vi "GeoCal_RangeWalk_process.vi"(0 "Position":string) -> (7 "Boolean":bool=TRUE)   [LabVIEW 2018]
panel:
  in  "Acquire":bool
  # "Geo Cal & Range Walk Test"
  # "please make sure the robot is in position\n                 then press the Acquire button"
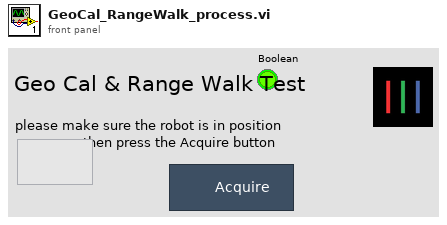
[diagram p1: front panel]
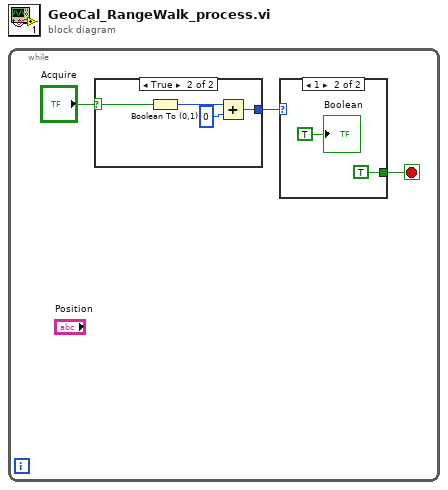
[diagram p0: block diagram]
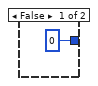
[diagram p2: hidden frame]
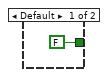
[diagram p3: hidden frame]
diagram:
  n1 = while {
    stop <- w3 stop-if-true
    n2 = case shown="True" "Acquire" {
      selector: "Acquire" -> [_ w5]
      tunnel: [i16 0 w6] -> w1
      frame False {
      }
      frame True {
        n3 = Boolean To (0,1)(Boolean=w5) -> (0, 1=w8:i16)
        n4 = Add(x=w8, y=i16 0) -> (x+y=w6:i16)
      }
    }
    n5 = case shown="1" w1 {
      tunnel: [FALSE TRUE] -> w3
      frame Default {
      }
      frame 1 {
        "Boolean" <- TRUE
      }
    }
  }
